vi "Analysator Betriebsdaten laden.vi"(10 "Analysator Definition":T1=[["NDIR lo", "CO", "ppm", "500", "2500", "10000", "1,2"], ["NDIR lo", "CO2", "ppm", "2000", "5000", "", "4,5"], ["NDIR hi", "CO", "%", "5", "", "", "6"], ["NDIR hi", "CO2", "%", "15", "30", "", "7"], ["PMA", "O2", "%", "25", "", "", "8"], ["FID", "HC", "ppm", "500", "2500", "10000", "9,10,11"]]) -> (2 "Betriebsdaten":T2[](array[typedef]))   [LabVIEW 2020, in "Analysator Definition.lvlib"]
uses:
  Analysator Definition.lvlib
  Betriebsdaten Komponente.ctl
  Analysator Definition.ctl
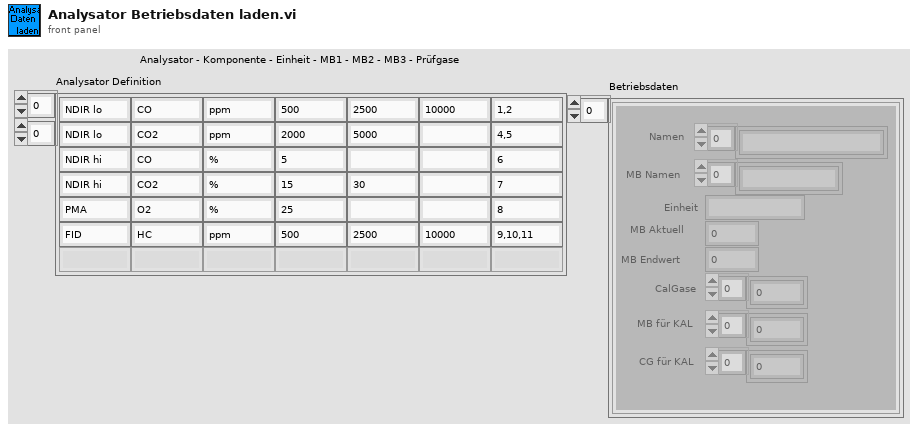
[diagram p1: front panel]
types:
  T1 = typedef "Analysator Definition.lvlib/Analysator Definition.ctl" = string[][]
  T2 = typedef "Analysator Definition.lvlib/Betriebsdaten Komponente.ctl" = cluster{"Namen":string[], "MB Namen":string[], "Einheit":string, "MB Aktuell":u16, "MB Endwert":u16, "CalGase":u16[], "MB für KAL":u16[], "CG für KAL":u16[]}
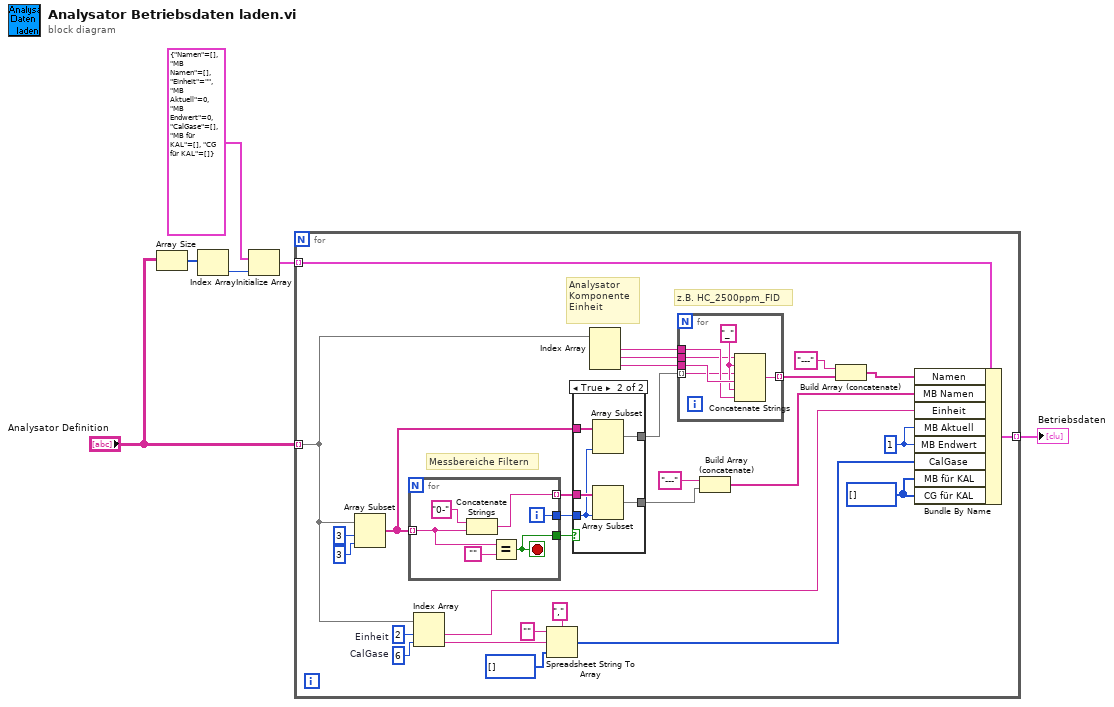
[diagram p0: block diagram]
diagram:
  n1 = Array Size(array="Analysator Definition") -> (size(s)=w6:i32[])
  n2 = Index Array(array=w6) -> (element=w5:i32)  [unwired: 1 in]
  n3 = Initialize Array(T2 {"Namen"=[], "MB Namen"=[], "Einheit"="", "MB Aktuell"=0, "MB Endwert"=0, "CalGase"=[], "MB für KAL"=[], "CG für KAL"=[]} ("Betreibsdaten Komponente"), w5) -> (w3:T2[])
  n4 = for {
    tunnel: "Analysator Definition" -> [w18] mode=indexing
    tunnel: w3 -> [w23] mode=indexing
    tunnel: [w17] -> w2 mode=indexing
    w8 = 2  # Einheit
    w11 = u16 1 ("MB Aktuell")
    w13 = u16[] [] ("MB für KAL")
    w10 = 6  # CalGase
    # "z.B. HC_2500ppm_FID"
    # "Analysator\nKomponente\nEinheit"
    # "Messbereiche Filtern"
    n5 = Array Subset(array=w18, index=3 ("Index"), length=3 ("Länge")) -> (w28:string[])
    n6 = for {
      tunnel: w28 -> [w50] mode=indexing
      tunnel: [w53] -> w33
      tunnel: [w52] -> w32
      tunnel: [w49] -> w29 mode=indexing
      i -> [w52]
      stop <- w53 stop-if-true
      n7 = Concatenate Strings("0-" ("String"), w50) -> (w49:string)
      n8 = Equal?(x=w50, y="") -> (x = y?=w53:bool)
    }
    n9 = Index Array(array=w18, index #1=w8, index #2=w10) -> (element #1=w7:string, element #2=w9:string)
    n10 = Spreadsheet String To Array(delimiter (Tab)="," ("Trennzeichen (Tabulator)"), format string="" ("Format-String"), spreadsheet string=w9, array type (2D Dbl)=u16[] []) -> (array=w12:u16[])
    n11 = case shown="True" w33 {
      tunnel: w29 -> [w43 w48]
      tunnel: w32 -> [_ w45]
      tunnel: [w43 w47] -> w30
      tunnel: w28 -> [w42 w46]
      tunnel: [w42 w44] -> w27
      frame False {
      }
      frame True {
        n12 = Array Subset(array=w46, length=w45) -> (w44:string[])  [unwired: 1 in]
        n13 = Array Subset(array=w48, length=w45) -> (w47:string[])  [unwired: 1 in]
      }
    }
    n14 = Index Array(array=w18) -> (element #1=w26:string, element #2=w25:string, element #3=w24:string)  [unwired: 3 in]
    n15 = for {
      tunnel: w27 -> [w37] mode=indexing
      tunnel: w26 -> [w40]
      tunnel: w25 -> [w38]
      tunnel: w24 -> [w41]
      tunnel: [w36] -> w15 mode=indexing
      w39 = "_"
      n16 = Concatenate Strings(w38, w39, w37, w41, w39, w40) -> (w36:string)
    }
    n17 = Build Array (concatenate)("---", w30) -> (w22:string[])
    n18 = Build Array (concatenate)("---", w15) -> (w14:string[])
    n19 = Bundle By Name(cluster=w23, "Namen"=w14, "MB Namen"=w22, "Einheit"=w7, "MB Aktuell"=w11, "MB Endwert"=w11, "CalGase"=w12, "MB für KAL"=w13, "CG für KAL"=w13) -> (w17:T2)
  }
  "Betriebsdaten" <- w2
